vi "Main.vi"(7 "sweep rate, /min":dbl=0.2, 8 "sweep to:":dbl=-0.5, 9 "sweep":T3(radio)=enum."time_sweep") -> ()   [LabVIEW 2017]
uses:
  controls/Channel.ctl
  controls/Measure.ctl
  controls/iPSreadCtrl.ctl
  controls/iTCreadCtrl.ctl
  controls/Source.ctl
  <vilib>/Utility/file.llb/Write To Spreadsheet File (DBL).vi
  <vilib>/gmath/NI_Gmath.lvlib
  <instrlib>/Keithley 2450/Keithley 2450.lvlib
  HULK SMS/SMScontrols.ctl
panel:
  in  "iTC_503_addr_sweep":u8=25
  in  "ITC503S addr_step":u8=24
  in  "IPS120-10 addr_Step":u8=25
  in  "IPS120-0 addr_sweep":u8=25
  out "DownNameString":string
  out "UpNameString":string
  in  "MappingName":string
  in  "Channel":T1=enum."b"
  in  "Mini steps":dbl=30.0
  in  "Tolerance_Step":dbl=0.01
  in  "Step Slope":dbl
  in  "Step Offset":dbl
  in  "diagonal step":bool
  in  "FieldRate(T/min)":dbl=0.1
  out "at field":bool
  in  "step":T2(radio)=enum."Radio Selection 6"
  in  "2336A_addr_step":refnum<visa-resource-name>="Keithley2614B"
  in  "2400_2_addr_step":u8=12
  in  "2400_1_addr_step":u8=12
  in  "wait between sweeps(s)":u32=1
  in  "Wait Between Step(s)":i32=1
  in  "Stop Mapping":bool
  in  "Start Mapping":bool
  in  "EstimateTime":bool
  out "MM:":dbl
  out "SS":dbl
  out "HH:":dbl
  out "Finish Time":timestamp
  out "Sweep Direction":string
  out "Current Step Value":dbl
  out "Table Index":dbl
  in  "Populate step table?":bool
  in  "Step values":string[][](table)=[["-20"], ["-10"], ["-4"], ["-1"], ["3"], ["6"], ["10"], [""]]
  in  "to":dbl=1.0
  in  "step":dbl=2.0
  in  "from":dbl=1.0
  in  "Cytec_Switch":bool
  in  "Lockin_Setup":bool
  in  "CH_A":bool
  in  "CH_B":bool
  in  "SR830 4 oop":bool
  in  "SR830 4 ip":bool
  in  "SR830 3 oop":bool
  in  "SR830 3 ip":bool
  in  "SR830 2 oop":bool
  in  "SR830 2 ip":bool
  in  "SR830 1 oop":bool
  in  "SR830 1 ip":bool
  in  "SR830 4 addr":u8=4
  in  "SR830 3 addr":u8=3
  in  "SR830 2 addr":u8=2
  in  "SR830 1 addr":u8=1
  in  "2182A 4 ch2":bool
  in  "2182A 4 ch1":bool
  in  "2182A 3 ch2":bool
  in  "2182A 3 ch1":bool
  in  "2182A 2 ch2":bool
  in  "2182A 2 ch1":bool
  in  "2182A 4 addr":u8=18
  in  "2182A 3 addr":u8=17
  in  "2182A 2 addr":u8=16
  in  "2182A 1 addr":u8=15
  in  "2182A 1 ch2":bool
  in  "2182A 1 ch1":bool
  in  "Tolerance_Sweep":dbl=0.01
  out "status 3":bool
  in  "Y_right_formula":string="brty/10/(300*10^-9)"
  in  "Yright":u16(ring)=3 caption="Y-Right:" items=["time_sweep", "time", "formula"]
  in  "Data Folder":path=path "C:/Users/b74305ys/Desktop/Research/DATA"
  out "Data file:":path=path "D:/Yanmeng/Data/Year2018/January2018/Jan2318/Jan2318x001.dat"
  out "status 2":bool
  in  "Show cursor":bool
  in  "Y_left_formula":string="brty/10/(300*10^-9)"
  in  "X_axis_formula":string
  in  "Yaxis":u16(ring)=3 caption="Y-Left:" items=["time_sweep", "time", "formula"]
  out "XY Graph":cluster{"Y Values":dbl[], "Y Values":dbl[]}[](graph)
  in  "Xaxis":u16(ring) caption="X-axis:" items=["time_sweep", "time", "formula"]
  out "status":bool
  in  "Initialize":bool
  in  "Quit":bool
  in  "Refresh Time(ms)":u32=100
  out "Sweep Channel":dbl
  out "Step Channel":dbl=-0.4901
  in  "Sweep Up":bool
  in  "Stop Ramp":bool
  in  "Up Rate":dbl
  in  "Down Rate":dbl
  in  "Ramp \nUp":bool
  in  "Ramp\n Down":bool
  in  "lower limit":dbl=-4.0
  in  "upper limit":dbl=4.0
  in  "Sweep Down":bool
  in  "Stop Sweep":bool
  in  "Continuous Sweep":bool
  in  "Slave Channel":T1=enum."b"
  in  "Double Sweep":bool
  in  "Slope":dbl
  in  "Offset":dbl
  in  "time/point, sec":dbl=0.5
  out "sweep value":dbl=2.186666666666735
  out "time delay, ms":dbl
  out "current time":timestamp=timestamp(3589630313.018 s since 1904-01-01) format="%<%H:%M:%S%1u>T"
  in  "iTC_Sample_T":bool
  in  "2400 3 addr":u8=14
  in  "2400 2 addr":u8=12
  in  "2400 1 addr":u8=12
  in  "2336A addr":refnum<visa-resource-name>="Keithley2614B"
  in  "sweep":bool
  in  "iPS_MagnetField":bool
  in  "auto\nrange B":bool
  in  "measure time":bool
  in  "2636A smub meas i":bool
  in  "2636A smub meas v":bool
  in  "2636A smua meas i":bool
  in  "2636A smua meas v":bool
  in  "2400 3 meas i":bool
  in  "2400 2 meas i":bool
  in  "2400 2 meas v":bool
  in  "2400 3 meas v":bool
  in  "2400 1 meas i":bool
  in  "2400 1 meas v":bool
  in  "auto\nrange A":bool
  in  "Monitor":bool
  in  "Linetrace or Mapping?":bool
  in  "Hulk_B_meas (Vnano)":bool
  in  "Hulk_SMS_addr":refnum<visa-resource-name>="TCPIP0::10.99.75.17::inst0::INSTR"
  in  "formula_variables":string[](array[string])=["a", "b", "c", "d", "e", "e", "f", "g", "h", "i", "j"]
  out "data":dbl[](array[numeric])
  out "Figure_axis":string[](array[string])=["HULK_SMS_output", "SR830_1_ip", "SR830_1_oop"]
  out "data_caption":string="HULK_SMS_output\tSR830_1_ip\tSR830_1_oop\t"
  # "Step Channel Setup"
  # "Sweep Channel Setup"
  # "SweepChannel"
  # "StepChannel"
  # "address"
  # "addres"
  # "2400_1"
  # "2400_2"
  # "2400_3"
  # "2636A_smua"
  # "2636A_smub"
  # "time"
  # "iPS"
  # "iTC"
  # "Teslatron iPS"
  # "Teslatron iTC"
  # "2400_1"
  # "2400_2"
  # "2636A_smua"
  # "2636A_smub"
  # "time"
  # "sweep"
  # "step"
  # "!Current sweep!"
  # "measure"
  # "MagnetField"
  # "Sample_T"
  # "voltage (_v)"
  # "current (_i)"
  # "Measure Channels"
  # "Lock-in amplifiers"
  # "Temp"
  # "address"
  # "Equipment"
  # "iTC"
  # "measure"
  # "SR830_1"
  # "SR830_2"
  # "SR830_3"
  # "SR830_4"
  # "in phase (_ip)"
  # "out of phase (_oop)"
  # "Nanovoltmeters"
  # "address"
  # "measure"
  # "2182A_1"
  # "2182A_2"
  # "2182A_3"
  # "2182A_4"
  # "channel 1 (_ch1)"
  # "channel 2 (_ch2)"
  # "(not recommended, slow)"
  # "Step Table"
  # "Current Value of Sweep and Step Channels"
  # "Sweep Parameters Setup"
  # "Down"
  # "Up"
  # "Limits"
  # "Rate\n(/min)"
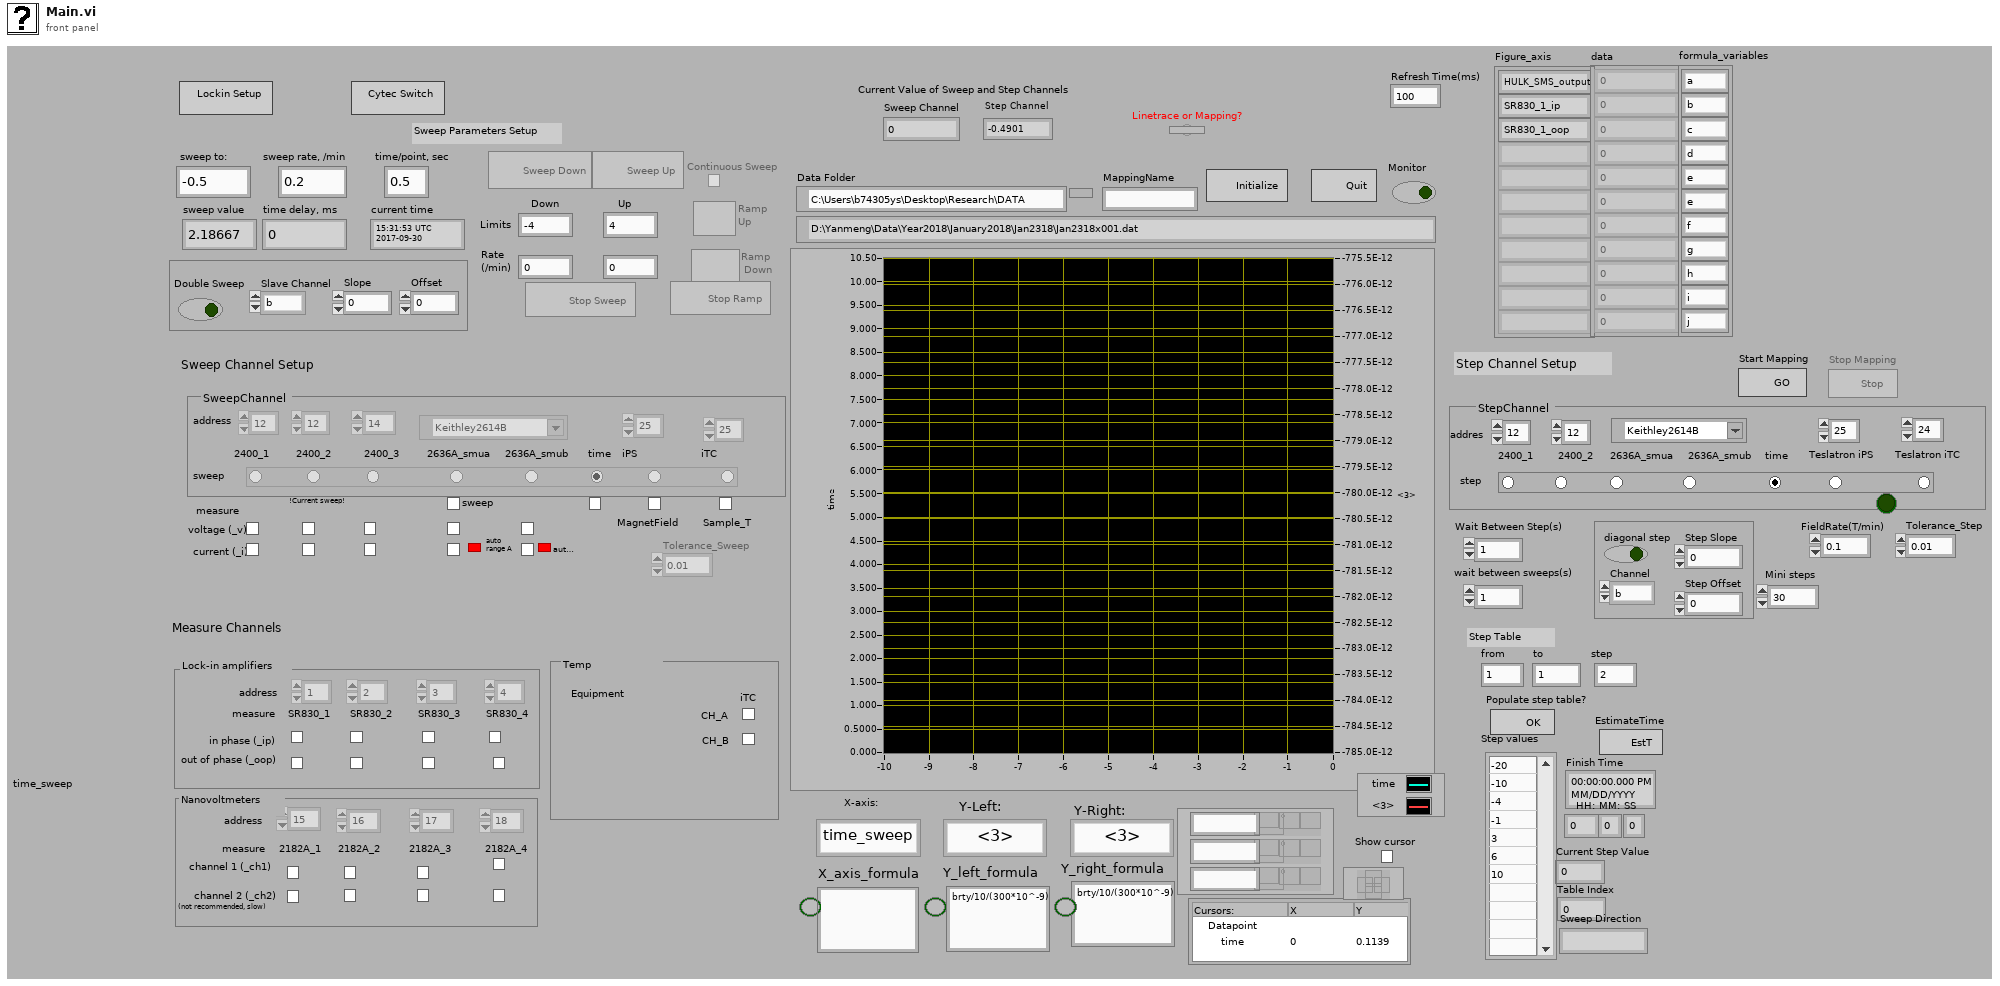
[diagram p1: front panel]
types:
  T1 = typedef "Channel.ctl" = enum16{"a", "b"}
  T2 = enum32{"Radio Selection 1", "Radio Selection 2", "Radio Selection 4", "Radio Selection 5", "Radio Selection 6", "Radio Selection 8", "Radio Selection 7"}
  T3 = enum32{"2400_1", "2400_2", "2400_3", "2636a_smua", "2636a_smub", "time_sweep", "iPS", "iTC"}
  T4 = cluster{"vi reference":refnum<vi>, "vi reference":refnum<vi>}
  T5 = enum8{"Enabled", "Disabled", "Disabled and Grayed Out"}
  T6 = typedef "Measure.ctl" = enum16{"Voltage", "Current", "Resistance", "Power"}
  T7 = typedef "SMScontrols.ctl" = enum16{"UPDATE", "GET OUTPUT", "RAMP ZERO", "RAMP MID", "RAMP MAX", "RAMP STATUS", "PAUSE OFF", "PAUSE ON", "HEATER OFF", "HEATER ON", "TESLA OFF", "TESLA ON", "DIRECTION +", "DIRECTION -", "DIRECTION 0", "SET MID", "SET MAX", "SET RAMP", "SET LIMIT", "SET TPA", "SET HEATER"}
  T8 = typedef "iPSreadCtrl.ctl" = enum16{"OutputField", "MagnetField", "Switch Heater Temp", "Field Rate", "Magnet Temp"}
  T9 = typedef "iTCreadCtrl.ctl" = enum16{"PT1 Temp", "PT2 Temp", "Sample Temp", "VTI Temp", "Needle Valve", "VTI Heater Power", "Sample Heater Power", "VTI Pressure"}
  T10 = typedef "Source.ctl" = enum16{"Current", "Voltage"}
  T11 = enum32{"Radio Selection 1", "Radio Selection 2", "Radio Selection 3", "Radio Selection 4", "Radio Selection 5", "Radio Selection 6", "Radio Selection 7"}
  T12 = enum32{"Bad", "Idle", "Run top level", "Running"}
diagram:
  # "This template is for the Producer/Consumer design pattern."
  # "initial value"
  n1 = flat-sequence {
    tunnel: [w15] -> w2
    tunnel: [w7] -> w1
    frame #0 {
      n2 = Current VI's Path() -> (path=w22:path)
      n3 = Strip Path(path=w22) -> (stripped path=w13:path)  [unwired: 1 out]
      n4 = Build Path(base path=w13, name or relative path="subVIs\\MagnetControl.vi") -> (appended path=w18:path)
      n5 = Build Path(base path=w13, name or relative path="subVIs\\TemperatureControl.vi") -> (appended path=w19:path)
      n6 = Build Path(base path=w13, name or relative path="subVIs\\CytecControl.vi") -> (appended path=w11:path)
      n7 = Build Path(base path=w13, name or relative path="subVIs\\Lockin Control Panel.vi") -> (appended path=w10:path)
      n8 = Open VI Reference(vi path=w18) -> (vi reference=w16:refnum<vi>)  [unwired: 5 in, 1 out]
      n9 = Open VI Reference(vi path=w19) -> (vi reference=w17:refnum<vi>)  [unwired: 5 in, 1 out]
      n10 = Open VI Reference(vi path=w10) -> (vi reference=w8:refnum<vi>)  [unwired: 5 in, 1 out]
      n11 = Open VI Reference(vi path=w11) -> (vi reference=w9:refnum<vi>)  [unwired: 5 in, 1 out]
      n12 = Bundle("vi reference"=w9, "vi reference"=w8) -> (w7:T4)  [unwired: 1 in]
      n13 = Bundle("vi reference"=w17, "vi reference"=w16) -> (w15:T4)  [unwired: 1 in]
    }
    frame #1 {
      w24 = T5."Disabled and Grayed Out" ("Disabled")
      w26 = T5."Enabled" ("Disabled")
      # "1 = 2400 1\n2 = 2400 2\n3 = 2400 3\n4 = 2636a smua\n5 = 2636a smub\n6 = do not sweep, just time\n7 = Magnetic Field IPS120\n8= 2461 smu"
      # "delete previous values"
      n14 = property on="Linetrace or Mapping?" class="Bool (strict)"() -> ("Value"=w25:bool)  [unwired: 2 in, 2 out]
      n15 = case shown="True" w25 {
        frame False {
          w29 = T5."Disabled and Grayed Out" ("Disabled")
          w30 = T5."Enabled" ("Disabled")
          n16 = property on="Tolerance_Sweep" class="DigNum (strict)"("DisabledEnum"=w30) -> ()  [unwired: 2 in, 2 out]
          n17 = property on="Ramp\n Down" class="Bool"("DisabledEnum"=w30) -> ()  [unwired: 2 in, 2 out]
          n18 = property on="IPS120-0 addr_sweep" class="DigNum (strict)"("DisabledEnum"=w30) -> ()  [unwired: 2 in, 2 out]
          n19 = property on="iTC_503_addr_sweep" class="DigNum (strict)"("DisabledEnum"=w30) -> ()  [unwired: 2 in, 2 out]
          n20 = property on="sweep" class="RadioBtnsControl (strict)"("DisabledEnum"=w30) -> ()  [unwired: 2 in, 2 out]
          n21 = property on="2182A 1 addr" class="DigNum (strict)"("DisabledEnum"=w30) -> ()  [unwired: 2 in, 2 out]
          n22 = property on="2182A 2 addr" class="DigNum (strict)"("DisabledEnum"=w30) -> ()  [unwired: 2 in, 2 out]
          n23 = property on="2182A 3 addr" class="DigNum (strict)"("DisabledEnum"=w30) -> ()  [unwired: 2 in, 2 out]
          n24 = property on="2182A 4 addr" class="DigNum (strict)"("DisabledEnum"=w30) -> ()  [unwired: 2 in, 2 out]
          n25 = property on="2400 1 addr" class="DigNum (strict)"("DisabledEnum"=w30) -> ()  [unwired: 2 in, 2 out]
          n26 = property on="Continuous Sweep" class="Bool (strict)"("DisabledEnum"=w30) -> ()  [unwired: 2 in, 2 out]
          n27 = property on="Sweep Down" class="Bool"("DisabledEnum"=w30) -> ()  [unwired: 2 in, 2 out]
          n28 = property on="Sweep Up" class="Bool"("DisabledEnum"=w30) -> ()  [unwired: 2 in, 2 out]
          n29 = property on="SR830 2 addr" class="DigNum (strict)"("DisabledEnum"=w30) -> ()  [unwired: 2 in, 2 out]
          n30 = property on="SR830 3 addr" class="DigNum (strict)"("DisabledEnum"=w30) -> ()  [unwired: 2 in, 2 out]
          n31 = property on="2400 2 addr" class="DigNum (strict)"("DisabledEnum"=w30) -> ()  [unwired: 2 in, 2 out]
          n32 = property on="2400 3 addr" class="DigNum (strict)"("DisabledEnum"=w30) -> ()  [unwired: 2 in, 2 out]
          n33 = property on="2336A addr" class="VISAName"("DisabledEnum"=w30) -> ()  [unwired: 2 in, 2 out]
          n34 = property on="SR830 1 addr" class="DigNum (strict)"("DisabledEnum"=w30) -> ()  [unwired: 2 in, 2 out]
          n35 = property on="SR830 4 addr" class="DigNum (strict)"("DisabledEnum"=w30) -> ()  [unwired: 2 in, 2 out]
          n36 = property on="Ramp \nUp" class="Bool"("DisabledEnum"=w30) -> ()  [unwired: 2 in, 2 out]
          n37 = property on="MappingName" class="Str"("Visible"=FALSE) -> ()  [unwired: 2 in, 2 out]
          n38 = property on="step" class="RadioBtnsControl (strict)"("DisabledEnum"=w29) -> ()  [unwired: 2 in, 2 out]
          n39 = property on="diagonal step" class="Bool (strict)"("DisabledEnum"=w29) -> ()  [unwired: 2 in, 2 out]
          n40 = property on="FieldRate(T/min)" class="DigNum (strict)"("DisabledEnum"=w29) -> ()  [unwired: 2 in, 2 out]
          n41 = property on="Step Offset" class="DigNum (strict)"("DisabledEnum"=w29) -> ()  [unwired: 2 in, 2 out]
          n42 = property on="Tolerance_Step" class="DigNum (strict)"("DisabledEnum"=w29) -> ()  [unwired: 2 in, 2 out]
          n43 = property on="Step Slope" class="DigNum (strict)"("DisabledEnum"=w29) -> ()  [unwired: 2 in, 2 out]
          n44 = property on="wait between sweeps(s)" class="DigNum (strict)"("DisabledEnum"=w29) -> ()  [unwired: 2 in, 2 out]
          n45 = property on="2336A_addr_step" class="VISAName"("DisabledEnum"=w29) -> ()  [unwired: 2 in, 2 out]
          n46 = property on="Start Mapping" class="Bool"("DisabledEnum"=w29) -> ()  [unwired: 2 in, 2 out]
          n47 = property on="2400_1_addr_step" class="DigNum (strict)"("DisabledEnum"=w29) -> ()  [unwired: 2 in, 2 out]
          n48 = property on="Wait Between Step(s)" class="DigNum (strict)"("DisabledEnum"=w29) -> ()  [unwired: 2 in, 2 out]
          n49 = property on="2400_2_addr_step" class="DigNum (strict)"("DisabledEnum"=w29) -> ()  [unwired: 2 in, 2 out]
          n50 = property on="IPS120-10 addr_Step" class="DigNum (strict)"("DisabledEnum"=w29) -> ()  [unwired: 2 in, 2 out]
          n51 = property on="ITC503S addr_step" class="DigNum (strict)"("DisabledEnum"=w29) -> ()  [unwired: 2 in, 2 out]
        }
        frame True {
          w33 = T5."Disabled and Grayed Out" ("Disabled")
          w32 = T5."Enabled" ("Disabled")
          n52 = property on="Ramp\n Down" class="Bool"("DisabledEnum"=w33) -> ()  [unwired: 2 in, 2 out]
          n53 = property on="sweep" class="RadioBtnsControl (strict)"("DisabledEnum"=w33) -> ()  [unwired: 2 in, 2 out]
          n54 = property on="2182A 1 addr" class="DigNum (strict)"("DisabledEnum"=w33) -> ()  [unwired: 2 in, 2 out]
          n55 = property on="2182A 2 addr" class="DigNum (strict)"("DisabledEnum"=w33) -> ()  [unwired: 2 in, 2 out]
          n56 = property on="2182A 3 addr" class="DigNum (strict)"("DisabledEnum"=w33) -> ()  [unwired: 2 in, 2 out]
          n57 = property on="2182A 4 addr" class="DigNum (strict)"("DisabledEnum"=w33) -> ()  [unwired: 2 in, 2 out]
          n58 = property on="2400 1 addr" class="DigNum (strict)"("DisabledEnum"=w33) -> ()  [unwired: 2 in, 2 out]
          n59 = property on="Tolerance_Sweep" class="DigNum (strict)"("DisabledEnum"=w33) -> ()  [unwired: 2 in, 2 out]
          n60 = property on="Sweep Down" class="Bool"("DisabledEnum"=w33) -> ()  [unwired: 2 in, 2 out]
          n61 = property on="SR830 2 addr" class="DigNum (strict)"("DisabledEnum"=w33) -> ()  [unwired: 2 in, 2 out]
          n62 = property on="SR830 3 addr" class="DigNum (strict)"("DisabledEnum"=w33) -> ()  [unwired: 2 in, 2 out]
          n63 = property on="2400 2 addr" class="DigNum (strict)"("DisabledEnum"=w33) -> ()  [unwired: 2 in, 2 out]
          n64 = property on="2400 3 addr" class="DigNum (strict)"("DisabledEnum"=w33) -> ()  [unwired: 2 in, 2 out]
          n65 = property on="2336A addr" class="VISAName"("DisabledEnum"=w33) -> ()  [unwired: 2 in, 2 out]
          n66 = property on="SR830 1 addr" class="DigNum (strict)"("DisabledEnum"=w33) -> ()  [unwired: 2 in, 2 out]
          n67 = property on="SR830 4 addr" class="DigNum (strict)"("DisabledEnum"=w33) -> ()  [unwired: 2 in, 2 out]
          n68 = property on="Ramp \nUp" class="Bool"("DisabledEnum"=w33) -> ()  [unwired: 2 in, 2 out]
          n69 = property on="IPS120-0 addr_sweep" class="DigNum (strict)"("DisabledEnum"=w33) -> ()  [unwired: 2 in, 2 out]
          n70 = property on="iTC_503_addr_sweep" class="DigNum (strict)"("DisabledEnum"=w33) -> ()  [unwired: 2 in, 2 out]
          n71 = property on="Continuous Sweep" class="Bool (strict)"("DisabledEnum"=w33) -> ()  [unwired: 2 in, 2 out]
          n72 = property on="Continuous Sweep" class="Bool (strict)"("Value"=FALSE ("Continuous Sweep")) -> ()  [unwired: 2 in, 2 out]
          n73 = property on="MappingName" class="Str"("Visible"=TRUE) -> ()  [unwired: 2 in, 2 out]
          n74 = property on="step" class="RadioBtnsControl (strict)"("DisabledEnum"=w32) -> ()  [unwired: 2 in, 2 out]
          n75 = property on="Step Offset" class="DigNum (strict)"("DisabledEnum"=w32) -> ()  [unwired: 2 in, 2 out]
          n76 = property on="diagonal step" class="Bool (strict)"("DisabledEnum"=w32) -> ()  [unwired: 2 in, 2 out]
          n77 = property on="Step Slope" class="DigNum (strict)"("DisabledEnum"=w32) -> ()  [unwired: 2 in, 2 out]
          n78 = property on="wait between sweeps(s)" class="DigNum (strict)"("DisabledEnum"=w32) -> ()  [unwired: 2 in, 2 out]
          n79 = property on="FieldRate(T/min)" class="DigNum (strict)"("DisabledEnum"=w32) -> ()  [unwired: 2 in, 2 out]
          n80 = property on="2336A_addr_step" class="VISAName"("DisabledEnum"=w32) -> ()  [unwired: 2 in, 2 out]
          n81 = property on="Start Mapping" class="Bool"("DisabledEnum"=w32) -> ()  [unwired: 2 in, 2 out]
          n82 = property on="2400_1_addr_step" class="DigNum (strict)"("DisabledEnum"=w32) -> ()  [unwired: 2 in, 2 out]
          n83 = property on="Wait Between Step(s)" class="DigNum (strict)"("DisabledEnum"=w32) -> ()  [unwired: 2 in, 2 out]
          n84 = property on="Tolerance_Step" class="DigNum (strict)"("DisabledEnum"=w32) -> ()  [unwired: 2 in, 2 out]
          n85 = property on="2400_2_addr_step" class="DigNum (strict)"("DisabledEnum"=w32) -> ()  [unwired: 2 in, 2 out]
          n86 = property on="IPS120-10 addr_Step" class="DigNum (strict)"("DisabledEnum"=w32) -> ()  [unwired: 2 in, 2 out]
          n87 = property on="ITC503S addr_step" class="DigNum (strict)"("DisabledEnum"=w32) -> ()  [unwired: 2 in, 2 out]
        }
      }
      n88 = property on="time delay, ms" class="DigNum (strict)"("Value"=u32 0 ("delib time delay")) -> ()  [unwired: 2 in, 2 out]
      n89 = local write "data"(dbl[] [] ("data")) -> ()
      n90 = property on="Monitor" class="Bool (strict)"() -> ("Value"=w23:bool)  [unwired: 2 in, 2 out]
      n91 = property on="formula_variables" class="Arr (strict)"("Visible"=w23) -> ()  [unwired: 2 in, 2 out]
      n92 = property on="data" class="Arr (strict)"("Visible"=w23) -> ()  [unwired: 2 in, 2 out]
      n93 = property on="Figure_axis" class="Arr (strict)"("Visible"=w23) -> ()  [unwired: 2 in, 2 out]
      n94 = property on="Stop Mapping" class="Bool"("DisabledEnum"=w24) -> ()  [unwired: 2 in, 2 out]
      n95 = property on="Stop Sweep" class="Bool"("DisabledEnum"=w24) -> ()  [unwired: 2 in, 2 out]
      n96 = property on="Stop Ramp" class="Bool"("DisabledEnum"=w24) -> ()  [unwired: 2 in, 2 out]
      n97 = property on="sweep" class="RadioBtnsControl (strict)"("DisabledEnum"=w26) -> ()  [unwired: 2 in, 2 out]
      n98 = property on="2182A 1 addr" class="DigNum (strict)"("DisabledEnum"=w26) -> ()  [unwired: 2 in, 2 out]
      n99 = property on="2182A 2 addr" class="DigNum (strict)"("DisabledEnum"=w26) -> ()  [unwired: 2 in, 2 out]
      n100 = property on="2182A 3 addr" class="DigNum (strict)"("DisabledEnum"=w26) -> ()  [unwired: 2 in, 2 out]
      n101 = property on="2182A 4 addr" class="DigNum (strict)"("DisabledEnum"=w26) -> ()  [unwired: 2 in, 2 out]
      n102 = property on="2400 1 addr" class="DigNum (strict)"("DisabledEnum"=w26) -> ()  [unwired: 2 in, 2 out]
      n103 = property on="SR830 2 addr" class="DigNum (strict)"("DisabledEnum"=w26) -> ()  [unwired: 2 in, 2 out]
      n104 = property on="SR830 3 addr" class="DigNum (strict)"("DisabledEnum"=w26) -> ()  [unwired: 2 in, 2 out]
      n105 = property on="2400 2 addr" class="DigNum (strict)"("DisabledEnum"=w26) -> ()  [unwired: 2 in, 2 out]
      n106 = property on="2400 3 addr" class="DigNum (strict)"("DisabledEnum"=w26) -> ()  [unwired: 2 in, 2 out]
      n107 = property on="2336A addr" class="VISAName"("DisabledEnum"=w26) -> ()  [unwired: 2 in, 2 out]
      n108 = property on="SR830 1 addr" class="DigNum (strict)"("DisabledEnum"=w26) -> ()  [unwired: 2 in, 2 out]
      n109 = property on="SR830 4 addr" class="DigNum (strict)"("DisabledEnum"=w26) -> ()  [unwired: 2 in, 2 out]
    }
  }
  n110 = Obtain Queue(name (unnamed)="Action", element data type="" ("data (can be any type)")) -> (queue out=w3:refnum<queue>)  [unwired: 3 in, 2 out]
  n111 = while {
    tunnel: [w38] -> w4
    tunnel: w3 -> [w36]
    stop <- w37 stop-if-true
    # "This loop is a consumer loop."
    n112 = Dequeue Element(queue=w36) -> (queue out=w38:refnum<queue>, element=w39:string)  [unwired: 2 in, 2 out]
    n113 = case shown="\"Ramp To Limit\"" w39 {
      tunnel: w38 -> [w40 _ _ w3851 _]
      tunnel: w38 -> [_ w1210 w2570 _ _]
      tunnel: [_ _ _ _ TRUE] -> w37
      frame "Idle", Default {
        # "0 = SR830_1_ip\n1 = SR830_1_oop\n2 = SR830_2_ip\n3 = SR830_2_oop\n4 = SR830_3_ip\n5 = SR830_3_oop\n6 = SR830_4_ip \n7 = SR830_4_oop \n8= 2400_1_v \n9 = 2400_1_i \n10 = 2400_2_v\n11 = 2400_2_i \n12 = 2400_3_v \n13 = 2400_3_i \n14 = 2182A_1_ch1 \n15 = 2182A_1_ch2 \n16 = 2182A_2_ch1 \n17 = 2182A_2_ch2\n18 = 2182A_3_ch1 \n19 = 2182A_3_ch2 \n20 = 2182A_4_ch1 \n21 = 2182A_4_ch2 \n22 = 2636A_smua_v \n23 = 2636A_smua_i \n24 = 2636A_smub_v \n25 = 2636A_smub_i \n26 = time\n27 = iPS_120\n28 = iTC _sample_T\n29= iTC _CH_A\n30=iTC_CH_B\n31 = Step_Value"
        n114 = stacked-sequence {
          tunnel: w40 -> [_ _ _ w1206]
          frame #0 {
            # "Read current value of sweep channel"
            # "1 = 2400 1\n2 = 2400 2\n3 = 2400 3\n4 = 2636a smua\n5 = 2636a smub\n6 = do not sweep, just time\n7 =IPS120-10\n8 =2461_smu"
            n115 = property on="sweep" class="RadioBtnsControl (strict)"() -> ("Value"=w42:T3)  [unwired: 2 in, 2 out]
            n116 = case "reads current value from instrument which will be sweeping" shown="\"iTC\"" w42 {
              tunnel: [w43 w53 w62 w71 w75 0.0 ("Measuremet") w80 w164] -> w41
              frame "2400_1", Default {
                # "reads the voltage on 2400 1"
                n117 = local read "2400 1 addr"() -> (w47:u8)
                n118 = Number To Decimal String(number=w47) -> (decimal integer string=w48:string)  [unwired: 1 in]
                n119 = GPIB Write(0:w48, 1:":READ?") -> (6:w44:errorcluster)  [unwired: 3 in, 1 out]
                n120 = GPIB Read(0:w48, 1:3200, 3:w44) -> (5:w50:string)  [unwired: 2 in, 2 out]
                n121 = String Subset(string=w50, length (rest)=13) -> (substring=w51:string)  [unwired: 1 in]
                n122 = Fract/Exp String To Number(string=w51) -> (number=w43:dbl)  [unwired: 3 in, 1 out]
              }
              frame "2400_2" {
                # "reads the current on 2400 2"
                n123 = local read "2400 2 addr"() -> (w57:u8)
                n124 = Number To Decimal String(number=w57) -> (decimal integer string=w58:string)  [unwired: 1 in]
                n125 = GPIB Write(0:w58, 1:":READ?") -> (6:w54:errorcluster)  [unwired: 3 in, 1 out]
                n126 = GPIB Read(0:w58, 1:3200, 3:w54) -> (5:w60:string)  [unwired: 2 in, 2 out]
                n127 = String Subset(string=w60, offset (0)=14, length (rest)=13) -> (substring=w61:string)
                n128 = Fract/Exp String To Number(string=w61) -> (number=w53:dbl)  [unwired: 3 in, 1 out]
              }
              frame "2400_3" {
                # "reads the voltage on 2400 3"
                n129 = local read "2400 3 addr"() -> (w66:u8)
                n130 = Number To Decimal String(number=w66) -> (decimal integer string=w67:string)  [unwired: 1 in]
                n131 = GPIB Write(0:w67, 1:":READ?") -> (6:w63:errorcluster)  [unwired: 3 in, 1 out]
                n132 = GPIB Read(0:w67, 1:3200, 3:w63) -> (5:w69:string)  [unwired: 2 in, 2 out]
                n133 = String Subset(string=w69, length (rest)=13) -> (substring=w70:string)  [unwired: 1 in]
                n134 = Fract/Exp String To Number(string=w70) -> (number=w62:dbl)  [unwired: 3 in, 1 out]
              }
              frame "2636a_smua" {
                # "reads the voltage on 2636a smua"
                n135 = local read "2336A addr"() -> (w74:refnum<visa-resource-name>)
                n136 = call "SinglePointMeasurement.vi"("Measure"=Measure."Voltage", "Channel"=Channel."a", "VISA resource name 2"=w74) -> ("Measuremet"=w71:dbl)  [unwired: 3 in, 4 out]
              }
              frame "2636a_smub" {
                # "reads the voltage on 2636a smub"
                n137 = local read "2336A addr"() -> (w78:refnum<visa-resource-name>)
                n138 = call "SinglePointMeasurement.vi"("Measure"=Measure."Voltage", "Channel"=Channel."b", "VISA resource name 2"=w78) -> ("Measuremet"=w75:dbl)  [unwired: 3 in, 4 out]
              }
              frame "time_sweep" {
              }
              frame "iPS" {
                n139 = disable-structure shown="Enabled" {
                  disable-tunnel: [w81 w157] -> w80
                  frame Disabled {
                    n140 = stacked-sequence {
                      tunnel: [_ _ _ _ _ _ _ w139 _] -> w81
                      frame #0 {
                        # "initialize interface of HULK SMS"
                        n141 = local read "Hulk_SMS_addr"() -> (w88:refnum<visa-resource-name>)
                        n142 = VISA Open(VISA resource name=w88) -> (VISA resource name=w87:refnum<visa-resource-name>, error out=w86:errorcluster)  [unwired: 4 in]
                        n143 = VISA Clear(VISA resource name=w87, error in (no error)=w86) -> (VISA resource name out=w84:refnum<visa-resource-name>, error out=w83:errorcluster)
                        n144 = property class="Instr"(reference=w84, error in=w83, "General Settings:Timeout Value"=u32 2000) -> (error out=w82:errorcluster)  [unwired: 1 out]
                        n145 = local write item#-1(w82) -> ()
                      }
                      frame #1 {
                        w89 = SMScontrols."UPDATE" ("SMS controls")
                        # "check intialization"
                        n146 = local read "Hulk_SMS_addr"() -> (w93:refnum<visa-resource-name>)
                        n147 = local read item#-1() -> (w92)
                        n148 = call "SMSsendCommand.vi"("HULK SMS address in"=w93, "SMS controls"=w89, "error in"=w92) -> ("HULK SMS address out"=w94:refnum<visa-resource-name>, "error out"=w95:errorcluster)  [unwired: 14 in, 1 out]
                        n149 = call "WaitRS232.vi"("error in"=w95, "delay[160 ms]"=u32 1000) -> ("error out"=w97:errorcluster)  [unwired: 1 in]
                        n150 = call "SMSread.vi"("HULK SMS address in"=w94, "SMS controls"=w89, "error in"=w97) -> ("read buffer"=w90:string, "error out"=w91:errorcluster)  [unwired: 11 in, 4 out]
                        n151 = local write item#-1(w90) -> ()
                        n152 = local write item#-1(w91) -> ()
                      }
                      frame #2 {
                        n153 = Wait (ms)(milliseconds to wait=u32 200) -> ()  [unwired: 1 out]
                      }
                      frame #3 {
                        w99 = SMScontrols."TESLA ON" ("SMS controls")
                        # "set units to tesla"
                        n154 = local read "Hulk_SMS_addr"() -> (w103:refnum<visa-resource-name>)
                        n155 = local read item#-1() -> (w102)
                        n156 = call "SMSsendCommand.vi"("HULK SMS address in"=w103, "SMS controls"=w99, "error in"=w102) -> ("HULK SMS address out"=w104:refnum<visa-resource-name>, "error out"=w105:errorcluster)  [unwired: 14 in, 1 out]
                        n157 = call "WaitRS232.vi"("error in"=w105, "delay[160 ms]"=u32 1000) -> ("error out"=w107:errorcluster)  [unwired: 1 in]
                        n158 = call "SMSread.vi"("HULK SMS address in"=w104, "SMS controls"=w99, "error in"=w107) -> ("read buffer"=w100:string, "error out"=w101:errorcluster)  [unwired: 11 in, 4 out]
                        n159 = local write item#-1(w100) -> ()
                        n160 = local write item#-1(w101) -> ()
                      }
                      frame #4 {
                        w108 = T5."Disabled and Grayed Out" ("Disabled")
                        # "sorry, no control of sweep rate and target\nvalue during sweeping\n\n!!! do not forget to reactivate it in the PAUSE mode!!!"
                      }
                      frame #5 {
                        w112 = SMScontrols."SET RAMP" ("SMS controls")
                        # "preparing HULK SMS!"
                        # "actual sweep rate"
                        # "1sec delay\nbecause HULK is not very bright"
                        # "sets sweep rate for HULK SMS"
                        n161 = local read item#-1() -> (w126)
                        n162 = local read "Hulk_SMS_addr"() -> (w125:refnum<visa-resource-name>)
                        n163 = local read item#-1() -> (w123)
                        n164 = call "SweepRateConversion.vi"("RAMP rate in"=w126, "T/min to A/s (True)"=TRUE) -> ("RAMP rate out"=w124:dbl)
                        n165 = call "SMSsendCommand.vi"("HULK SMS address in"=w125, "SMS controls"=w112, "error in"=w123, "RAMP rate"=w124) -> ("HULK SMS address out"=w119:refnum<visa-resource-name>, "error out"=w120:errorcluster)  [unwired: 13 in, 1 out]
                        n166 = call "WaitRS232.vi"("error in"=w120, "delay[160 ms]"=u32 1000) -> ("error out"=w122:errorcluster)  [unwired: 1 in]
                        n167 = call "SMSread.vi"("HULK SMS address in"=w119, "SMS controls"=w112, "error in"=w122) -> ("read buffer"=w115:string, "error out"=w116:errorcluster)  [unwired: 11 in, 4 out]
                        n168 = Match Pattern(string=w115, regular expression="RAMP RATE:") -> (after substring=w118:string)  [unwired: 1 in, 3 out]
                        n169 = local write item#-1(w115) -> ()
                        n170 = Scan From String(format string="%.f", input string=w118, error in=w116) -> (error out=w113:errorcluster, output 1=w111:dbl)  [unwired: 2 in, 2 out]
                        n171 = local write item#-1(w113) -> ()
                        n172 = call "SweepRateConversion.vi"("RAMP rate in"=w111, "T/min to A/s (True)"=FALSE) -> ("RAMP rate out"=w109:dbl)
                        n173 = local write item#-1(w109) -> ()
                      }
                      frame #6 {
                        w128 = SMScontrols."SET MID" ("SMS controls")
                        # "sets target value for B field sweep"
                        n174 = local read "Hulk_SMS_addr"() -> (w131:refnum<visa-resource-name>)
                        n175 = local read item#-1() -> (w132)
                        n176 = local read item#-1() -> (w130)
                        n177 = call "SMSsendCommand.vi"("HULK SMS address in"=w131, "SMS controls"=w128, "error in"=w132, "MID field value"=w130) -> ("HULK SMS address out"=w136:refnum<visa-resource-name>, "error out"=w134:errorcluster)  [unwired: 13 in, 1 out]
                        n178 = call "WaitRS232.vi"("error in"=w134, "delay[160 ms]"=u32 1000) -> ("error out"=w135:errorcluster)  [unwired: 1 in]
                        n179 = call "SMSread.vi"("HULK SMS address in"=w136, "SMS controls"=w128, "error in"=w135) -> ("read buffer"=w129:string, "error out"=w133:errorcluster)  [unwired: 11 in, 4 out]
                        n180 = local write item#-1(w133) -> ()
                        n181 = local write item#-1(w129) -> ()
                      }
                      frame #7 {
                        # "acquires current output value"
                        n182 = local read "Hulk_SMS_addr"() -> (w142:refnum<visa-resource-name>)
                        n183 = local read item#-1() -> (w141)
                        n184 = call "SMS_GET_OUTPUT.vi"("CRYogenic:("=w141, "Hulk_SMS_addr"=w142) -> ("error IO"=w138:errorcluster, "read buffer"=w140:string, "Numeric"=w139:dbl)
                        n185 = local write item#-1(w138) -> ()
                        n186 = local write item#-1(w140) -> ()
                      }
                      frame #8 {
                        # "activates ramping"
                        n187 = local read item#-1() -> (w150)
                        n188 = Equal?(x=w150, y=0.0) -> (x = y?=w148:bool)
                        n189 = Select(t=SMScontrols."RAMP ZERO" ("SMS controls"), s=w148, f=SMScontrols."RAMP MID" ("SMS controls")) -> (s? t:f=w145:T7)
                        n190 = local read "Hulk_SMS_addr"() -> (w152:refnum<visa-resource-name>)
                        n191 = local read item#-1() -> (w151)
                        n192 = call "SMSsendCommand.vi"("HULK SMS address in"=w152, "SMS controls"=w145, "error in"=w151) -> ("HULK SMS address out"=w155:refnum<visa-resource-name>, "error out"=w154:errorcluster)  [unwired: 14 in, 1 out]
                        n193 = call "WaitRS232.vi"("error in"=w154, "delay[160 ms]"=u32 1000) -> ("error out"=w156:errorcluster)  [unwired: 1 in]
                        n194 = call "SMSread.vi"("HULK SMS address in"=w155, "SMS controls"=w145, "error in"=w156) -> ("read buffer"=w143:string, "error out"=w144:errorcluster)  [unwired: 11 in, 4 out]
                        n195 = local write item#-1(w144) -> ()
                        n196 = local write item#-1(w143) -> ()
                      }
                    }
                  }
                  frame Enabled {
                    w159 = 1
                    # "preparing Teslatron_iPS_Field"
                    # "Measure magnetic field on Teslatron_iPS_Field"
                    n197 = local read "IPS120-0 addr_sweep"() -> (w163:u8)
                    n198 = Number To Decimal String(number=w163) -> (decimal integer string=w162:string)  [unwired: 1 in]
                    n199 = GPIB Write(0:w162, 1:"R 7", 2:w159) -> ()  [unwired: 2 in, 2 out]
                    n200 = GPIB Read(0:w162, 1:200 ("byte count"), 2:w159) -> (5:w161:string)  [unwired: 2 in, 2 out]
                    n201 = Fract/Exp String To Number(string=w161, offset=w159) -> (number=w157:dbl)  [unwired: 2 in, 1 out]
                  }
                }
              }
              frame "iTC" {
                n202 = disable-structure shown="Enabled" {
                  disable-tunnel: [w172 w179] -> w164
                  frame Disabled {
                    w175 = u16 0 items=["Volts", "Current", "Auto Resistance", "Manual Resistance", "Digitize Voltage", "Digitize Current"] ("Function (0: Volts)")
                    w169 = u16 1 items=["Volts", "Current"] ("Function (0: Volts)")
                    n203 = call <instrlib>:"Configure Source Limit Level.vi"("Source Limit (1.0)"=5.0, "Function (0: Volts)"=w169) -> ("error out"=w167:errorcluster, "VISA resource name out"=w170:refnum<visa-resource-name>, "VISA resource name"=w171:refnum<visa-resource-name>)  [unwired: 7 in]
                    n204 = call <instrlib>:"Configure Measurement Function.vi"("error in (no error)"=w167, "Function (0: Volts)"=w175, "VISA resource name"=w170) -> ("error out"=w166:errorcluster, "VISA resource name out"=w174:refnum<visa-resource-name>)  [unwired: 7 in]
                    n205 = call <instrlib>:"Enable Output.vi"("error in (no error)"=w166, "VISA resource name"=w174) -> ("error out"=w165:errorcluster, "VISA resource name out"=w173:refnum<visa-resource-name>)  [unwired: 8 in]
                    n206 = call <instrlib>:"Get Source Level.vi"("error in (no error)"=w165, "VISA resource name"=w173) -> ("Current Level Out"=w172:dbl)  [unwired: 6 in, 3 out]
                  }
                  frame Enabled {
                    w178 = i16 1 ("mode (0)")
                    (unwired) 1
                    # "temporarily ITC503S"
                    n207 = property on="iTC_503_addr_sweep" class="DigNum (strict)"() -> ("Value"=w181:u8)  [unwired: 2 in, 2 out]
                    n208 = Number To Decimal String(number=w181) -> (decimal integer string=w182:string)  [unwired: 1 in]
                    n209 = GPIB Write(0:w182, 1:"$C3") -> (6:w183:errorcluster)  [unwired: 3 in, 1 out]
                    n210 = GPIB Write(0:w182, 1:"R3", 2:w178, 3:w183) -> (6:w185:errorcluster)  [unwired: 1 in, 1 out]
                    n211 = GPIB Read(0:w182, 1:200, 2:w178, 3:w185) -> (5:w184:string)  [unwired: 1 in, 2 out]
                    n212 = Fract/Exp String To Number(string=w184, offset=w178) -> (number=w179:dbl)  [unwired: 2 in, 1 out]
                  }
                }
              }
            }
            n213 = property on="Sweep Channel" class="DigNum (strict)"("Value"=w41) -> ()  [unwired: 2 in, 2 out]
          }
          frame #1 {
            # "Read Current value of step channel"
            n214 = property on="Linetrace or Mapping?" class="Bool (strict)"() -> ("Value"=w186:bool)  [unwired: 2 in, 2 out]
            n215 = case shown="True" w186 {
              frame False {
                n216 = property on="Step Channel" class="DigNum (strict)"("Value"=9999999.0 ("Step Channel")) -> ()  [unwired: 2 in, 2 out]
              }
              frame True {
                # "1 = 2400 1\n2 = 2400 2\n3 = 2400 3\n4 = 2636a smua\n5 = 2636a smub\n6 = do not sweep, just time\n7 =IPS120-10\n8 =2461_smu"
                n217 = property on="step" class="RadioBtnsControl (strict)"() -> ("Value"=w189:T2)  [unwired: 2 in, 2 out]
                n218 = case "reads current value from instrument which will be stepping" shown="\"Radio Selection 8\"" w189 {
                  tunnel: [w191 w201 w210 w214 0.0 ("Measuremet") w218 w227] -> w188
                  frame "Radio Selection 1", Default {
                    # "reads the voltage on 2400 1"
                    n219 = property on="2400_1_addr_step" class="DigNum (strict)"() -> ("Value"=w190:u8)  [unwired: 2 in, 2 out]
                    n220 = Number To Decimal String(number=w190) -> (decimal integer string=w195:string)  [unwired: 1 in]
                    n221 = GPIB Write(0:w195, 1:":READ?") -> (6:w192:errorcluster)  [unwired: 3 in, 1 out]
                    n222 = GPIB Read(0:w195, 1:3200, 3:w192) -> (5:w197:string)  [unwired: 2 in, 2 out]
                    n223 = String Subset(string=w197, length (rest)=13) -> (substring=w198:string)  [unwired: 1 in]
                    n224 = Fract/Exp String To Number(string=w198) -> (number=w191:dbl)  [unwired: 3 in, 1 out]
                  }
                  frame "Radio Selection 2" {
                    # "reads the current on 2400 2"
                    n225 = property on="2400_2_addr_step" class="DigNum (strict)"() -> ("Value"=w199:u8)  [unwired: 2 in, 2 out]
                    n226 = Number To Decimal String(number=w199) -> (decimal integer string=w205:string)  [unwired: 1 in]
                    n227 = GPIB Write(0:w205, 1:":READ?") -> (6:w202:errorcluster)  [unwired: 3 in, 1 out]
                    n228 = GPIB Read(0:w205, 1:3200, 3:w202) -> (5:w207:string)  [unwired: 2 in, 2 out]
                    n229 = String Subset(string=w207, offset (0)=14, length (rest)=13) -> (substring=w208:string)
                    n230 = Fract/Exp String To Number(string=w208) -> (number=w201:dbl)  [unwired: 3 in, 1 out]
                  }
                  frame "Radio Selection 4" {
                    # "reads the voltage on 2636a smua"
                    n231 = property on="2336A_addr_step" class="VISAName"() -> ("Value"=w209:refnum<visa-resource-name>)  [unwired: 2 in, 2 out]
                    n232 = call "SinglePointMeasurement.vi"("Measure"=Measure."Voltage", "Channel"=Channel."a", "VISA resource name 2"=w209) -> ("Measuremet"=w210:dbl)  [unwired: 3 in, 4 out]
                  }
                  frame "Radio Selection 5" {
                    # "reads the voltage on 2636a smub"
                    n233 = property on="2336A_addr_step" class="VISAName"() -> ("Value"=w213:refnum<visa-resource-name>)  [unwired: 2 in, 2 out]
                    n234 = call "SinglePointMeasurement.vi"("Measure"=Measure."Voltage", "Channel"=Channel."b", "VISA resource name 2"=w213) -> ("Measuremet"=w214:dbl)  [unwired: 3 in, 4 out]
                  }
                  frame "Radio Selection 6" {
                  }
                  frame "Radio Selection 7" {
                    w220 = 1
                    # "Measure magnetic field on IPS"
                    n235 = local read "IPS120-10 addr_Step"() -> (w224:u8)
                    n236 = Number To Decimal String(number=w224) -> (decimal integer string=w223:string)  [unwired: 1 in]
                    n237 = GPIB Write(0:w223, 1:"R 7", 2:w220) -> ()  [unwired: 2 in, 2 out]
                    n238 = GPIB Read(0:w223, 1:200 ("byte count"), 2:w220) -> (5:w222:string)  [unwired: 2 in, 2 out]
                    n239 = Fract/Exp String To Number(string=w222, offset=w220) -> (number=w218:dbl)  [unwired: 2 in, 1 out]
                  }
                  frame "Radio Selection 8" {
                    w226 = 1
                    # "temporarily ITC503S"
                    n240 = property on="ITC503S addr_step" class="DigNum (strict)"() -> ("Value"=w225:u8)  [unwired: 2 in, 2 out]
                    n241 = Number To Decimal String(number=w225) -> (decimal integer string=w232:string)  [unwired: 1 in]
                    n242 = GPIB Write(0:w232, 1:"$C3", 2:1) -> (6:w233:errorcluster)  [unwired: 2 in, 1 out]
                    n243 = GPIB Write(0:w232, 1:"R3", 2:w226, 3:w233) -> (6:w235:errorcluster)  [unwired: 1 in, 1 out]
                    n244 = GPIB Read(0:w232, 1:200, 2:w226, 3:w235) -> (5:w234:string)  [unwired: 1 in, 2 out]
                    n245 = Fract/Exp String To Number(string=w234, offset=w226) -> (number=w227:dbl)  [unwired: 2 in, 1 out]
                  }
                }
                n246 = property on="Step Channel" class="DigNum (strict)"("Value"=w188) -> ()  [unwired: 2 in, 2 out]
              }
            }
          }
          frame #2 {
            # "Update current value of measured channel"
            n247 = property on="Monitor" class="Bool (strict)"() -> ("Value"=w236:bool)  [unwired: 2 in, 2 out]
            n248 = case shown="True" w236 {
              frame False {
              }
              frame True {
                n249 = stacked-sequence {
                  frame #0 {
                    # "Prepare the display format"
                    n250 = local read "2636A smua meas v"() -> (w242:bool)
                    n251 = local read "2636A smub meas v"() -> (w240:bool)
                    n252 = local read "2636A smub meas i"() -> (w239:bool)
                    n253 = local read "2636A smua meas i"() -> (w241:bool)
                    n254 = property on="sweep" class="RadioBtnsControl (strict)"() -> ("Value"=w237:T3)  [unwired: 2 in, 2 out]
                    n255 = Compound Arithmetic op=OR(w242, w241, w240, w239) -> (w238:bool)
                    n256 = case shown="True" w238 {
                      frame False {
                      }
                      frame True {
                        # "opens session for 2636a system sourcemeter"
                        n257 = local read "2336A addr"() -> (w291:refnum<visa-resource-name>)
                        n258 = VISA Close(VISA resource name=w291) -> ()  [unwired: 1 in, 1 out]
                      }
                    }
                    n259 = case shown="\"iTC\"" w237 {
                      frame "2400_1" {
                        # "add label for the first column in the datafile"
                        n260 = stacked-sequence {
                          frame #0 {
                            n261 = property on="data_caption" class="Str"("Value"="") -> ()  [unwired: 2 in, 2 out]
                            n262 = property on="Figure_axis" class="Arr (strict)"("Value"=string[] [] ("Figure_axis_string")) -> ()  [unwired: 2 in, 2 out]
                          }
                          frame #1 {
                            w245 = "V_sweep_2400_1" ("V_sweep")
                            n263 = Concatenate Strings(w245, "\t") -> (w247:string)
                            n264 = Build Array(w245) -> (w246:string[])
                            n265 = property on="data_caption" class="Str"("Value"=w247) -> ()  [unwired: 2 in, 2 out]
                            n266 = property on="Figure_axis" class="Arr (strict)"("Value"=w246) -> ()  [unwired: 2 in, 2 out]
                          }
                        }
                      }
                      frame "2400_2" {
                        n267 = stacked-sequence {
                          frame #0 {
                            n268 = property on="data_caption" class="Str"("Value"="") -> ()  [unwired: 2 in, 2 out]
                            n269 = property on="Figure_axis" class="Arr (strict)"("Value"=string[] [] ("Figure_axis_string")) -> ()  [unwired: 2 in, 2 out]
                          }
                          frame #1 {
                            w251 = "V_sweep_2400_2" ("V_sweep")
                            n270 = Build Array(w251) -> (w252:string[])
                            n271 = Concatenate Strings(w251, "\t") -> (w254:string)
                            n272 = property on="Figure_axis" class="Arr (strict)"("Value"=w252) -> ()  [unwired: 2 in, 2 out]
                            n273 = property on="data_caption" class="Str"("Value"=w254) -> ()  [unwired: 2 in, 2 out]
                          }
                        }
                      }
                      frame "2400_3" {
                        n274 = stacked-sequence {
                          frame #0 {
                            n275 = property on="data_caption" class="Str"("Value"="") -> ()  [unwired: 2 in, 2 out]
                            n276 = property on="Figure_axis" class="Arr (strict)"("Value"=string[] [] ("Figure_axis_string")) -> ()  [unwired: 2 in, 2 out]
                          }
                          frame #1 {
                            w257 = "V_sweep_2400_3" ("V_sweep")
                            n277 = Concatenate Strings(w257, "\t") -> (w260:string)
                            n278 = Build Array(w257) -> (w258:string[])
                            n279 = property on="data_caption" class="Str"("Value"=w260) -> ()  [unwired: 2 in, 2 out]
                            n280 = property on="Figure_axis" class="Arr (strict)"("Value"=w258) -> ()  [unwired: 2 in, 2 out]
                          }
                        }
                      }
                      frame "2636a_smua" {
                        n281 = stacked-sequence {
                          frame #0 {
                            n282 = property on="data_caption" class="Str"("Value"="") -> ()  [unwired: 2 in, 2 out]
                            n283 = property on="Figure_axis" class="Arr (strict)"("Value"=string[] [] ("Figure_axis_string")) -> ()  [unwired: 2 in, 2 out]
                          }
                          frame #1 {
                            w263 = "V_sweep_2636a_smua" ("V_sweep")
                            n284 = Concatenate Strings(w263, "\t") -> (w266:string)
                            n285 = Build Array(w263) -> (w264:string[])
                            n286 = property on="data_caption" class="Str"("Value"=w266) -> ()  [unwired: 2 in, 2 out]
                            n287 = property on="Figure_axis" class="Arr (strict)"("Value"=w264) -> ()  [unwired: 2 in, 2 out]
                          }
                        }
                      }
                      frame "2636a_smub" {
                        n288 = stacked-sequence {
                          frame #0 {
                            n289 = property on="data_caption" class="Str"("Value"="") -> ()  [unwired: 2 in, 2 out]
                            n290 = property on="Figure_axis" class="Arr (strict)"("Value"=string[] [] ("Figure_axis_string")) -> ()  [unwired: 2 in, 2 out]
                          }
                          frame #1 {
                            w269 = "V_sweep_2636a_smub" ("V_sweep")
                            n291 = Build Array(w269) -> (w270:string[])
                            n292 = Concatenate Strings(w269, "\t") -> (w272:string)
                            n293 = property on="Figure_axis" class="Arr (strict)"("Value"=w270) -> ()  [unwired: 2 in, 2 out]
                            n294 = property on="data_caption" class="Str"("Value"=w272) -> ()  [unwired: 2 in, 2 out]
                          }
                        }
                      }
                      frame "time_sweep", Default {
                        n295 = stacked-sequence {
                          frame #0 {
                            n296 = property on="data_caption" class="Str"("Value"="") -> ()  [unwired: 2 in, 2 out]
                            n297 = property on="Figure_axis" class="Arr (strict)"("Value"=string[] [] ("Figure_axis_string")) -> ()  [unwired: 2 in, 2 out]
                          }
                          frame #1 {
                            w275 = "time_sweep" ("V_sweep")
                            n298 = Build Array(w275) -> (w276:string[])
                            n299 = Concatenate Strings(w275, "\t") -> (w277:string)
                            n300 = property on="Figure_axis" class="Arr (strict)"("Value"=w276) -> ()  [unwired: 2 in, 2 out]
                            n301 = property on="data_caption" class="Str"("Value"=w277) -> ()  [unwired: 2 in, 2 out]
                          }
                        }
                      }
                      frame "iPS" {
                        # "sweep iPS"
                        n302 = stacked-sequence {
                          frame #0 {
                            n303 = property on="data_caption" class="Str"("Value"="") -> ()  [unwired: 2 in, 2 out]
                            n304 = property on="Figure_axis" class="Arr (strict)"("Value"=string[] [] ("Figure_axis_string")) -> ()  [unwired: 2 in, 2 out]
                          }
                          frame #1 {
                            w281 = "iPS_OutputField" ("V_sweep")
                            n305 = Build Array(w281) -> (w282:string[])
                            n306 = Concatenate Strings(w281, "\t") -> (w284:string)
                            n307 = property on="Figure_axis" class="Arr (strict)"("Value"=w282) -> ()  [unwired: 2 in, 2 out]
                            n308 = property on="data_caption" class="Str"("Value"=w284) -> ()  [unwired: 2 in, 2 out]
                          }
                        }
                      }
                      frame "iTC" {
                        n309 = stacked-sequence {
                          frame #0 {
                            n310 = property on="data_caption" class="Str"("Value"="") -> ()  [unwired: 2 in, 2 out]
                            n311 = property on="Figure_axis" class="Arr (strict)"("Value"=string[] ["", "SR830_1_ip", "SR830_1_oop", "SR830_2_ip", "SR830_2_oop", "2461_meas_v", "2461_meas_i", "2636A_smua_v", "2636A_smua_i", "formula"] ("Figure_axis")) -> ()  [unwired: 2 in, 2 out]
                          }
                          frame #1 {
                            w289 = "iTC_sample"
                            n312 = Build Array(w289) -> (w288:string[])
                            n313 = Concatenate Strings(w289, "\t") -> (w287:string)
                            n314 = property on="data_caption" class="Str"("Value"=w287) -> ()  [unwired: 2 in, 2 out]
                            n315 = property on="Figure_axis" class="Arr (strict)"("Value"=w288) -> ()  [unwired: 2 in, 2 out]
                          }
                        }
                      }
                    }
                  }
                  frame #1 {
                    # "0 = SR830_1_ip\n1 = SR830_1_oop\n2 = SR830_2_ip\n3 = SR830_2_oop\n4 = SR830_3_ip\n5 = SR830_3_oop\n6 = SR830_4_ip \n7 = SR830_4_oop \n8= 2400_1_v \n9 = 2400_1_i \n10 = 2400_2_v\n11 = 2400_2_i \n12 = 2400_3_v \n13 = 2400_3_i \n14 = 2182A_1_ch1 \n15 = 2182A_1_ch2 \n16 = 2182A_2_ch1 \n17 = 2182A_2_ch2\n18 = 2182A_3_ch1 \n19 = 2182A_3_ch2 \n20 = 2182A_4_ch1 \n21 = 2182A_4_ch2 \n22 = 2636A_smua_v \n23 = 2636A_smua_i \n24 = 2636A_smub_v \n25 = 2636A_smub_i \n26 = time\n27 = iPS_120\n28 = iTC _sample_T\n29 = iTC _CH_A\n30=iTC_CH_B\n31 = Step_Value"
                    # "this part constructs the first (text) line for the data file with names of all measured variables,\nalso constructs a text array contaning names of all measured variable for the \"ring\" (so parameter can be selected and plotted)"
                    n316 = stacked-sequence {
                      frame #0 {
                        # "SR830 1 in phase (SR830_1_ip)"
                        n317 = local read "SR830 1 ip"() -> (w296:bool)
                        n318 = property on="Figure_axis" class="Arr (strict)"() -> ("Value"=w293:string[])  [unwired: 2 in, 2 out]
                        n319 = property on="data_caption" class="Str"() -> ("Value"=w295:string)  [unwired: 2 in, 2 out]
                        n320 = case shown="True" w296 {
                          tunnel: w295 -> [w298 w304]
                          tunnel: [w298 w303] -> w294
                          tunnel: w293 -> [w297 w301]
                          tunnel: [w297 w299] -> w292
                          frame False {
                            # "not measure SR830 1 in phase signal (SR830_1_ip)"
                          }
                          frame True {
                            w300 = "SR830_1_ip"
                            # "measure SR830 1 in phase signal (SR830_1_ip)"
                            n321 = local read "SR830 1 addr"() -> (w305:u8)
                            n322 = Number To Decimal String(number=w305) -> (decimal integer string=w306:string)  [unwired: 1 in]
                            n323 = GPIB Clear(3:w306) -> ()  [unwired: 1 in, 2 out]
                            n324 = Build Array (concatenate)(w301, w300) -> (w299:string[])
                            n325 = Concatenate Strings(w304, w300, "\t") -> (w303:string)
                          }
                        }
                        n326 = property on="Figure_axis" class="Arr (strict)"("Value"=w292) -> ()  [unwired: 2 in, 2 out]
                        n327 = property on="data_caption" class="Str"("Value"=w294) -> ()  [unwired: 2 in, 2 out]
                      }
                      frame #1 {
                        # "SR830 1 out of phase (SR830_1_oop)"
                        n328 = local read "SR830 1 oop"() -> (w311:bool)
                        n329 = property on="Figure_axis" class="Arr (strict)"() -> ("Value"=w308:string[])  [unwired: 2 in, 2 out]
                        n330 = property on="data_caption" class="Str"() -> ("Value"=w310:string)  [unwired: 2 in, 2 out]
                        n331 = case shown="False" w311 {
                          tunnel: w310 -> [w313 w319]
                          tunnel: [w313 w318] -> w309
                          tunnel: w308 -> [w312 w316]
                          tunnel: [w312 w314] -> w307
                          frame False {
                            # "not measure SR830 1 out of phase signal (SR830_1_oop)"
                          }
                          frame True {
                            w315 = "SR830_1_oop"
                            # "measure SR830 1 out of phase signal (SR830_1_oop)"
                            n332 = local read "SR830 1 addr"() -> (w320:u8)
                            n333 = Number To Decimal String(number=w320) -> (decimal integer string=w321:string)  [unwired: 1 in]
                            n334 = GPIB Clear(3:w321) -> ()  [unwired: 1 in, 2 out]
                            n335 = Build Array (concatenate)(w316, w315) -> (w314:string[])
                            n336 = Concatenate Strings(w319, w315, "\t") -> (w318:string)
                          }
                        }
                        n337 = property on="Figure_axis" class="Arr (strict)"("Value"=w307) -> ()  [unwired: 2 in, 2 out]
                        n338 = property on="data_caption" class="Str"("Value"=w309) -> ()  [unwired: 2 in, 2 out]
                      }
                      frame #2 {
                        # "SR830 2 in phase (SR830_2_ip)"
                        n339 = local read "SR830 2 ip"() -> (w326:bool)
                        n340 = property on="Figure_axis" class="Arr (strict)"() -> ("Value"=w323:string[])  [unwired: 2 in, 2 out]
                        n341 = property on="data_caption" class="Str"() -> ("Value"=w325:string)  [unwired: 2 in, 2 out]
                        n342 = case shown="True" w326 {
                          tunnel: w325 -> [w328 w334]
                          tunnel: [w328 w333] -> w324
                          tunnel: w323 -> [w327 w331]
                          tunnel: [w327 w329] -> w322
                          frame False {
                            # "not measure SR830 2 in phase signal (SR830_2_ip)"
                          }
                          frame True {
                            w330 = "SR830_2_ip"
                            # "measure SR830 2 in phase signal (SR830_2_ip)"
                            n343 = local read "SR830 2 addr"() -> (w335:u8)
                            n344 = Number To Decimal String(number=w335) -> (decimal integer string=w336:string)  [unwired: 1 in]
                            n345 = GPIB Clear(3:w336) -> ()  [unwired: 1 in, 2 out]
                            n346 = Build Array (concatenate)(w331, w330) -> (w329:string[])
                            n347 = Concatenate Strings(w334, w330, "\t") -> (w333:string)
                          }
                        }
                        n348 = property on="Figure_axis" class="Arr (strict)"("Value"=w322) -> ()  [unwired: 2 in, 2 out]
                        n349 = property on="data_caption" class="Str"("Value"=w324) -> ()  [unwired: 2 in, 2 out]
                      }
                      frame #3 {
                        # "SR830 2 out of phase (SR830_2_oop)"
                        n350 = local read "SR830 2 oop"() -> (w341:bool)
                        n351 = property on="Figure_axis" class="Arr (strict)"() -> ("Value"=w338:string[])  [unwired: 2 in, 2 out]
                        n352 = property on="data_caption" class="Str"() -> ("Value"=w340:string)  [unwired: 2 in, 2 out]
                        n353 = case shown="True" w341 {
                          tunnel: w340 -> [w343 w349]
                          tunnel: [w343 w348] -> w339
                          tunnel: w338 -> [w342 w346]
                          tunnel: [w342 w344] -> w337
                          frame False {
                            # "not measure SR830 2 out of phase signal (SR830_2_oop)"
                          }
                          frame True {
                            w345 = "SR830_2_oop"
                            # "measure SR830 2 out of phase signal (SR830_2_oop)"
                            n354 = local read "SR830 2 addr"() -> (w350:u8)
                            n355 = Number To Decimal String(number=w350) -> (decimal integer string=w351:string)  [unwired: 1 in]
                            n356 = GPIB Clear(3:w351) -> ()  [unwired: 1 in, 2 out]
                            n357 = Build Array (concatenate)(w346, w345) -> (w344:string[])
                            n358 = Concatenate Strings(w349, w345, "\t") -> (w348:string)
                          }
                        }
                        n359 = property on="Figure_axis" class="Arr (strict)"("Value"=w337) -> ()  [unwired: 2 in, 2 out]
                        n360 = property on="data_caption" class="Str"("Value"=w339) -> ()  [unwired: 2 in, 2 out]
                      }
                      frame #4 {
                        # "SR830 3 in phase (SR830_3_ip)"
                        n361 = local read "SR830 3 ip"() -> (w356:bool)
                        n362 = property on="Figure_axis" class="Arr (strict)"() -> ("Value"=w353:string[])  [unwired: 2 in, 2 out]
                        n363 = property on="data_caption" class="Str"() -> ("Value"=w355:string)  [unwired: 2 in, 2 out]
                        n364 = case shown="True" w356 {
                          tunnel: w355 -> [w358 w364]
                          tunnel: [w358 w363] -> w354
                          tunnel: w353 -> [w357 w361]
                          tunnel: [w357 w359] -> w352
                          frame False {
                            # "not measure SR830 3 in phase signal (SR830_3_ip)"
                          }
                          frame True {
                            w360 = "SR830_3_ip"
                            # "measure SR830 3 in phase signal (SR830_3_ip)"
                            n365 = local read "SR830 3 addr"() -> (w365:u8)
                            n366 = Number To Decimal String(number=w365) -> (decimal integer string=w366:string)  [unwired: 1 in]
                            n367 = GPIB Clear(3:w366) -> ()  [unwired: 1 in, 2 out]
                            n368 = Build Array (concatenate)(w361, w360) -> (w359:string[])
                            n369 = Concatenate Strings(w364, w360, "\t") -> (w363:string)
                          }
                        }
                        n370 = property on="Figure_axis" class="Arr (strict)"("Value"=w352) -> ()  [unwired: 2 in, 2 out]
                        n371 = property on="data_caption" class="Str"("Value"=w354) -> ()  [unwired: 2 in, 2 out]
                      }
                      frame #5 {
                        # "SR830 3 out of phase (SR830_3_oop)"
                        n372 = local read "SR830 3 oop"() -> (w371:bool)
                        n373 = property on="Figure_axis" class="Arr (strict)"() -> ("Value"=w368:string[])  [unwired: 2 in, 2 out]
                        n374 = property on="data_caption" class="Str"() -> ("Value"=w370:string)  [unwired: 2 in, 2 out]
                        n375 = case shown="True" w371 {
                          tunnel: w370 -> [w373 w379]
                          tunnel: [w373 w378] -> w369
